vi "Remember_value.vi"(1 "Mode":T1, 2 "Input Value":dbl format="%.2f", 3 "Ch name":string) -> (0 "Output Value":dbl format="%.2f")   [LabVIEW 2010]
uses:
  ADAM Controls/Remember_value_mode.ctl
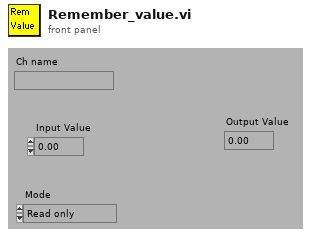
[diagram p1: front panel]
types:
  T1 = typedef "Remember_value_mode.ctl" = enum16{"Read only", "Read and Write"}
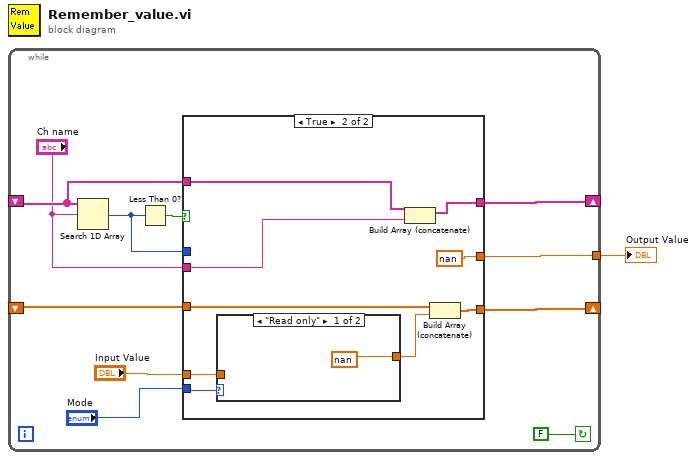
[diagram p0: block diagram]
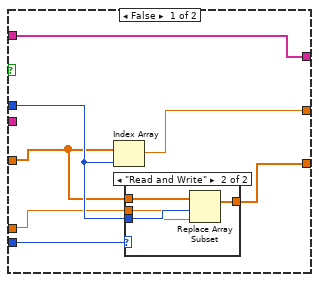
[diagram p2: hidden frame]
diagram:
  n1 = while {
    tunnel: [w4] -> w1
    shift-left: _ -> [w7]
    shift-right: [w6] -> _
    shift-left: _ -> [w11]
    shift-right: [w10] -> _
    stop <- FALSE continue-if-true
    n2 = Search 1D Array(1D array=w11, element="Ch name") -> (index of element=w8:i32)  [unwired: 1 out]
    n3 = Less Than 0?(x=w8) -> (x < 0?=w12:bool)
    n4 = case shown="True" w12 {
      tunnel: w11 -> [w19 w33]
      tunnel: [w19 w32] -> w10
      tunnel: "Ch name" -> [_ w31]
      tunnel: w8 -> [w18 _]
      tunnel: w7 -> [w17 w30]
      tunnel: [w15 w29] -> w6
      tunnel: "Input Value" -> [w16 w25]
      tunnel: [w14 nan ("Input Value")] -> w4
      tunnel: "Mode" -> [w13 w27]
      frame False {
        n5 = Index Array(array=w17, index=w18) -> (element=w14:dbl)
        n6 = case shown="\"Read and Write\"" w13 {
          tunnel: w18 -> [_ w24]
          tunnel: w17 -> [w20 w23]
          tunnel: w16 -> [_ w22]
          tunnel: [w20 w21] -> w15
          frame "Read only" {
          }
          frame "Read and Write" {
            n7 = Replace Array Subset(array=w23, new element=w22, index=w24) -> (w21:dbl[])
          }
        }
      }
      frame True {
        n8 = case shown="\"Read only\"" w27 {
          tunnel: [nan ("Input Value") w35] -> w26
          tunnel: w25 -> [_ w35]
          frame "Read only" {
          }
          frame "Read and Write" {
          }
        }
        n9 = Build Array (concatenate)(w33, w31) -> (w32:string[])
        n10 = Build Array (concatenate)(w30, w26) -> (w29:dbl[])
      }
    }
  }
  "Output Value" <- w1
